vi "getSerializedData.vi"(0 "reference in":refnum<class "DQMHModuleNode.lvclass">, 5 "error in (no error)":errorcluster) -> (14 "reference out":refnum<class "DQMHModuleNode.lvclass">, 15 "parent":refnum<class "AbstractNode.lvclass">, 16 "children":refnum<class "AbstractNode.lvclass">[](array[class]), 17 "xmlOut":string, 19 "error out":errorcluster)   [LabVIEW 2014, in "DQMHModuleNode.lvclass"]
doc: "Gets data to store"
uses:
  <resource>/Framework/Providers/Open_GDS/UML/DQMHModuleNode_class/DQMHModuleNode.lvclass
  <resource>/Framework/Providers/Open_GDS/UML/AbstractNode_class/AbstractNode.lvclass
  <resource>/Framework/Providers/Open_GDS/UML/MultiLineString_class/MultiLineString.lvclass
  <resource>/Framework/Providers/Open_GDS/UML/RectangularNode_class/RectangularNode.lvclass
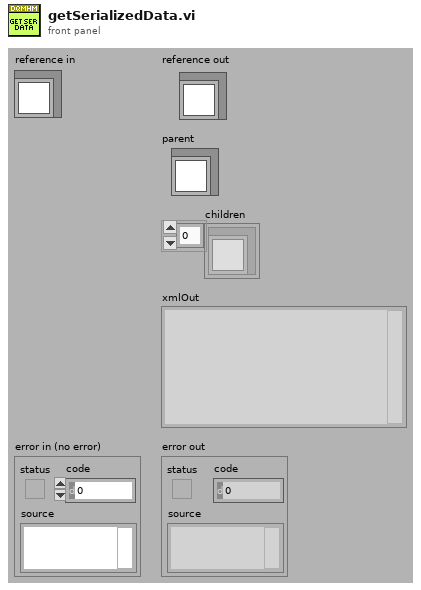
[diagram p1: front panel]
types:
  T1 = typedef "AbstractNode.lvclass/ObjectAttributes.ctl" = cluster{"parent":refnum<class "AbstractNode.lvclass">, "children":refnum<class "AbstractNode.lvclass">[], "Hidden":bool}
  T2 = typedef "RectangularNode.lvclass/ObjectAttributes.ctl" = cluster{"bounds":T3}
  T3 = typedef "Rectangle Rectangle2D.ctl" = cluster{"x":dbl, "y":dbl, "width":dbl, "height":dbl}
  T4 = typedef "DQMHModuleNode.lvclass/ObjectAttributes.ctl" = cluster{"midHeight":dbl, "botHeight":dbl, "Name":refnum<class "MultiLineString.lvclass">, "Description":refnum<class "MultiLineString.lvclass">, "InternalData":refnum<class "MultiLineString.lvclass">, "Events":refnum<class "MultiLineString.lvclass">, "DEFAULT_COMPARTMENT_HEIGHT":i32, "DEFAULT_WIDTH":i32, "DEFAULT_HEIGHT":i32, "showEvents":bool, "showInternalData":bool, "ClassPath":path, "Template":string, "Icon":u8[][]}
  T5 = cluster{cluster{"Data":T1, "Data":T2, "Data":T4}, "text":string, "text":string, "text":string, "text":string}
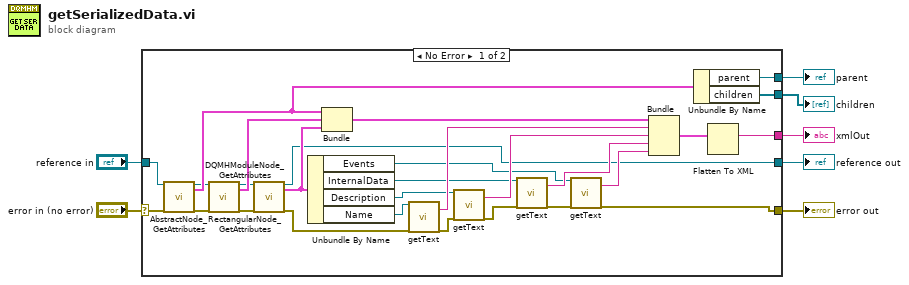
[diagram p0: block diagram]
diagram:
  n1 = case shown="No Error" "error in (no error)" {
    selector: "error in (no error)" -> [w13 w36]
    tunnel: "reference in" -> [w12 w37]
    tunnel: [w25 w36] -> w5
    tunnel: [w8 w37] -> w4
    tunnel: [w35 _] -> w3
    tunnel: [w34 _] -> w2
    tunnel: [w33 _] -> w1
    frame No Error {
      n2 = call <resource>:"AbstractNode_GetAttributes.vi"("reference in"=w12, "error in (no error)"=w13) -> ("reference out"=w10:refnum<class "DQMHModuleNode.lvclass">, "Data"=w19:T1, "error out"=w14:errorcluster)  [unwired: 14 in, 1 out]
      n3 = call <resource>:"RectangularNode_GetAttributes.vi"("reference in"=w10, "error in (no error)"=w14) -> ("reference out"=w11:refnum<class "DQMHModuleNode.lvclass">, "Data"=w18:T2, "error out"=w15:errorcluster)  [unwired: 14 in, 1 out]
      n4 = call <resource>:"DQMHModuleNode_GetAttributes.vi"("reference in"=w11, "error in (no error)"=w15) -> ("reference out"=w8:refnum<class "DQMHModuleNode.lvclass">, "Data"=w17:T4, "error out"=w9:errorcluster)  [unwired: 1 in, 14 out]
      n5 = Unbundle By Name(w17) -> ("Events"=w21:refnum<class "MultiLineString.lvclass">, "InternalData"=w22:refnum<class "MultiLineString.lvclass">, "Description"=w23:refnum<class "MultiLineString.lvclass">, "Name"=w24:refnum<class "MultiLineString.lvclass">)
      n6 = Bundle("Data"=w19, "Data"=w18, "Data"=w17) -> (w16:cluster{"Data":T1, "Data":T2, "Data":T4})  [unwired: 1 in]
      n7 = call-dynamic "getText.vi"("reference"=w24, "error in (no error)"=w9) -> ("text"=w29:string, "error out"=w30:errorcluster)  [unwired: 16 out]
      n8 = call-dynamic "getText.vi"("reference"=w23, "error in (no error)"=w30) -> ("text"=w28:string, "error out"=w31:errorcluster)  [unwired: 16 out]
      n9 = call-dynamic "getText.vi"("reference"=w22, "error in (no error)"=w31) -> ("text"=w27:string, "error out"=w26:errorcluster)  [unwired: 16 out]
      n10 = call-dynamic "getText.vi"("reference"=w21, "error in (no error)"=w26) -> ("text"=w20:string, "error out"=w25:errorcluster)  [unwired: 16 out]
      n11 = Bundle(w16, "text"=w29, "text"=w28, "text"=w27, "text"=w20) -> (w32:T5)  [unwired: 1 out]
      n12 = Unbundle By Name(w19) -> ("parent"=w35:refnum<class "AbstractNode.lvclass">, "children"=w34:refnum<class "AbstractNode.lvclass">[])
      n13 = Flatten To XML(anything=w32) -> (xml string=w33:string)
    }
    frame Error {
    }
  }
  "reference out" <- w4
  "error out" <- w5
  "children" <- w2
  "parent" <- w3
  "xmlOut" <- w1
